vi "mapPubDataSVToUE.vi"(6 "Time Stamp":timestamp, 8 "error in (no error)":errorcluster, 9 "svValue":variant, 10 "svArrayIndex":i32, 11 "MiddlewareSVThisComponent in":refnum<class "MiddlewareSVThisComponent.lvclass">) -> (0 "error out":errorcluster, 3 "MiddlewareSVThisComponent out":refnum<class "MiddlewareSVThisComponent.lvclass">)   [LabVIEW 2015, in "MiddlewareSVThisComponent.lvclass"]
uses:
  MiddlewareSVThisComponent.lvclass
  MiddlewareSVThisComponent.lvclass/MiddlewareSVThisComponent.ctl
  PubSubDataEvent/PubSubDataEvent.lvclass/PubSubDataEvent.ctl
  Typedefs/StateValue.ctl
  Typedefs/RejectedCommand.ctl
  Typedefs/CommandValue.ctl
  ComponentTemplateCore/ComponentModel/ComponentModel/Typedefs/ComponentStateValues.ctl
  PubSubDataEvent/PubSubDataEvent.lvclass
  Typedefs/EXATypedefs.lvlib
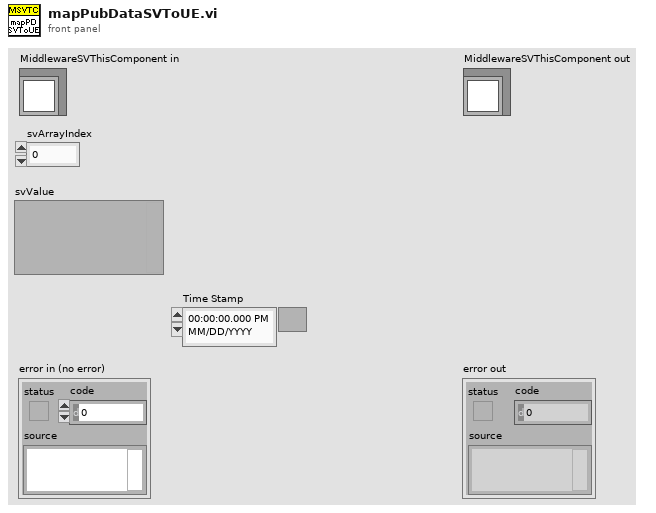
[diagram p1: front panel]
types:
  T1 = typedef "EXATypedefs.lvlib/PubDataSV.ctl" = enum16{"DetailedState", "ErrorCode", "Heartbeat", "LoopTime_ms", "LoopTimeOutOfRange", "RejectedCommand", "SummaryState", "Timestamp"}
  T2 = typedef "EXATypedefs.lvlib/PubDataEvents.ctl" = cluster{"DetailedState":refnum<user-event>, "ErrorCode":refnum<user-event>, "Heartbeat":refnum<user-event>, "LoopTime_ms":refnum<user-event>, "LoopTimeOutOfRange":refnum<user-event>, "RejectedCommand":refnum<user-event>, "SummaryState":refnum<user-event>, "Timestamp":refnum<user-event>}
  T3 = typedef "EXATypedefs.lvlib/StateValue.ctl" = enum16{"DisabledState", "EnabledState", "FaultState", "OffState", "StandbyState"}
  T4 = typedef "EXATypedefs.lvlib/RejectedCommand.ctl" = cluster{"CommandValue":T5, "StateValue":T3, "Time Stamp":timestamp}
  T5 = typedef "EXATypedefs.lvlib/CommandValue.ctl" = enum16{"ClearError", "Disable", "Enable", "Exit", "GoToStandby", "OnHeartbeat", "OnIncomingMessagingError", "OnInterrupt", "Start"}
  T6 = typedef "ComponentStateValues.ctl" = enum16{"Off", "Standby", "Enabled", "Disabled", "Fault"}
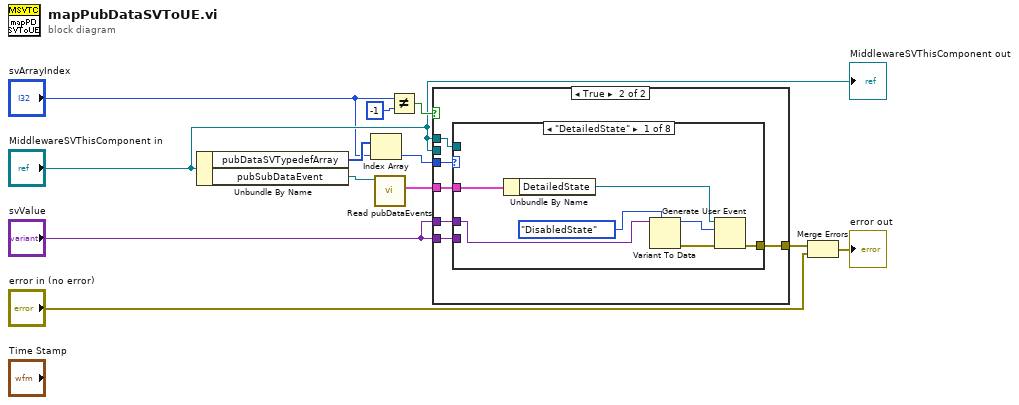
[diagram p0: block diagram]
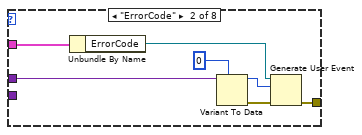
[diagram p3: hidden frame]
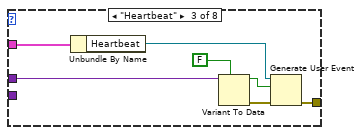
[diagram p4: hidden frame]
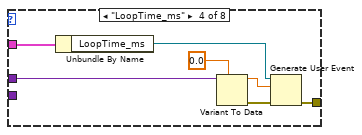
[diagram p5: hidden frame]
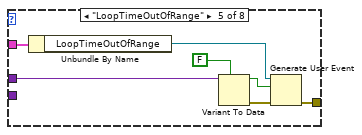
[diagram p6: hidden frame]
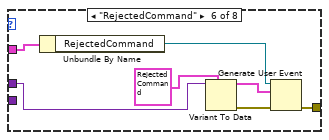
[diagram p7: hidden frame]
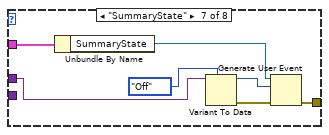
[diagram p8: hidden frame]
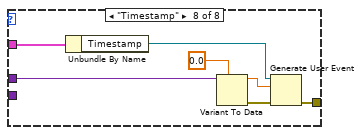
[diagram p9: hidden frame]
diagram:
  n1 = Unbundle By Name("MiddlewareSVThisComponent in") -> ("pubDataSVTypedefArray"=w12:T1[], "pubSubDataEvent"=w2:refnum<class "PubSubDataEvent.lvclass">)
  n2 = Index Array(array=w12, index="svArrayIndex") -> (element=w10:T1)
  n3 = call "Read pubDataEvents.vi"("PubSubDataEvent in"=w2) -> ("pubDataEvents"=w1:T2)  [unwired: 9 in, 1 out]
  n4 = Not Equal?(x="svArrayIndex", y=-1) -> (x != y?=w8:bool)
  n5 = case shown="True" w8 {
    tunnel: "svValue" -> [_ w15]
    tunnel: [_ w18] -> w11
    tunnel: w10 -> [_ w17]
    tunnel: "MiddlewareSVThisComponent in" -> [_ _]
    tunnel: w1 -> [_ w16]
    tunnel: "MiddlewareSVThisComponent in" -> [_ w14]
    tunnel: "svValue" -> [_ w13]
    frame False {
    }
    frame True {
      n6 = case shown="\"DetailedState\"" w17 {
        tunnel: w15 -> [w23 w30 w38 w44 w52 w58 w65 w72]
        tunnel: [w19 w26 w33 w40 w47 w54 w61 w68] -> w18
        tunnel: w16 -> [w25 w32 w39 w46 w53 w60 w67 w74]
        tunnel: w14 -> [_ _ _ _ _ _ _ _]
        tunnel: w13 -> [_ _ _ _ _ _ _ _]
        frame "DetailedState" {
          n7 = Unbundle By Name(w25) -> ("DetailedState"=w24:refnum<user-event>)
          n8 = Variant To Data(type=StateValue."DisabledState" ("event data"), Variant=w23) -> (data=w21:T3, error out=w20:errorcluster)  [unwired: 1 in]
          n9 = Generate User Event(user event=w24, event data cluster=w21, error in=w20) -> (error out=w19:errorcluster)  [unwired: 1 in, 1 out]
        }
        frame "ErrorCode" {
          n10 = Unbundle By Name(w32) -> ("ErrorCode"=w31:refnum<user-event>)
          n11 = Variant To Data(type=0 ("event data"), Variant=w30) -> (data=w28:i32, error out=w27:errorcluster)  [unwired: 1 in]
          n12 = Generate User Event(user event=w31, event data cluster=w28, error in=w27) -> (error out=w26:errorcluster)  [unwired: 1 in, 1 out]
        }
        frame "Heartbeat" {
          n13 = Unbundle By Name(w39) -> ("Heartbeat"=w37:refnum<user-event>)
          n14 = Variant To Data(type=FALSE ("event data"), Variant=w38) -> (data=w35:bool, error out=w34:errorcluster)  [unwired: 1 in]
          n15 = Generate User Event(user event=w37, event data cluster=w35, error in=w34) -> (error out=w33:errorcluster)  [unwired: 1 in, 1 out]
        }
        frame "LoopTime_ms" {
          n16 = Unbundle By Name(w46) -> ("LoopTime_ms"=w45:refnum<user-event>)
          n17 = Variant To Data(type=0.0 ("event data"), Variant=w44) -> (data=w42:dbl, error out=w41:errorcluster)  [unwired: 1 in]
          n18 = Generate User Event(user event=w45, event data cluster=w42, error in=w41) -> (error out=w40:errorcluster)  [unwired: 1 in, 1 out]
        }
        frame "LoopTimeOutOfRange" {
          n19 = Unbundle By Name(w53) -> ("LoopTimeOutOfRange"=w51:refnum<user-event>)
          n20 = Variant To Data(type=FALSE ("event data"), Variant=w52) -> (data=w49:bool, error out=w48:errorcluster)  [unwired: 1 in]
          n21 = Generate User Event(user event=w51, event data cluster=w49, error in=w48) -> (error out=w47:errorcluster)  [unwired: 1 in, 1 out]
        }
        frame "RejectedCommand" {
          n22 = Unbundle By Name(w60) -> ("RejectedCommand"=w59:refnum<user-event>)
          n23 = Variant To Data(type=T4 {"CommandValue"=enum."ClearError", "StateValue"=enum."DisabledState", "Time Stamp"=timestamp(0 s since 1904-01-01)} ("event data"), Variant=w58) -> (data=w56:T4, error out=w55:errorcluster)  [unwired: 1 in]
          n24 = Generate User Event(user event=w59, event data cluster=w56, error in=w55) -> (error out=w54:errorcluster)  [unwired: 1 in, 1 out]
        }
        frame "SummaryState" {
          n25 = Unbundle By Name(w67) -> ("SummaryState"=w66:refnum<user-event>)
          n26 = Variant To Data(type=ComponentStateValues."Off" ("event data"), Variant=w65) -> (data=w63:T6, error out=w62:errorcluster)  [unwired: 1 in]
          n27 = Generate User Event(user event=w66, event data cluster=w63, error in=w62) -> (error out=w61:errorcluster)  [unwired: 1 in, 1 out]
        }
        frame "Timestamp" {
          n28 = Unbundle By Name(w74) -> ("Timestamp"=w73:refnum<user-event>)
          n29 = Variant To Data(type=0.0 ("event data"), Variant=w72) -> (data=w70:dbl, error out=w69:errorcluster)  [unwired: 1 in]
          n30 = Generate User Event(user event=w73, event data cluster=w70, error in=w69) -> (error out=w68:errorcluster)  [unwired: 1 in, 1 out]
        }
      }
    }
  }
  n31 = Merge Errors(w11, "error in (no error)") -> (→"error out":errorcluster)
  "MiddlewareSVThisComponent out" <- "MiddlewareSVThisComponent in"
